vi "GlobalGraphTwo7.vi"(2 "1D Names Input Array":string[](array[string]), 3 "Cluster Array Input":cluster{"Array":dbl[], "Array 2":dbl[]}[](array[cluster]), 4 "Graph Select":dbl, 5 "Function select":string) -> (0 "1D Names Output Array":string[](array[string]), 1 "Cluster Array Output":cluster{"Array":dbl[], "Array 2":dbl[]}[](array[cluster]))   [LabVIEW 2015]
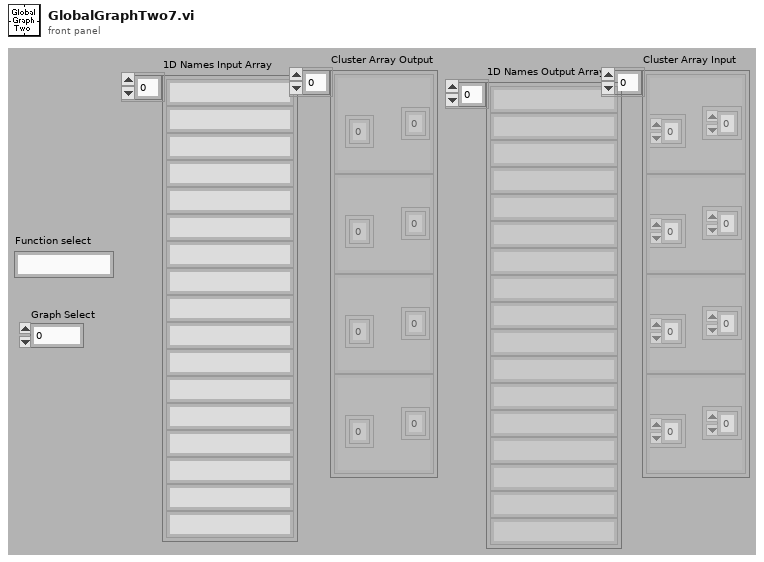
[diagram p1: front panel]
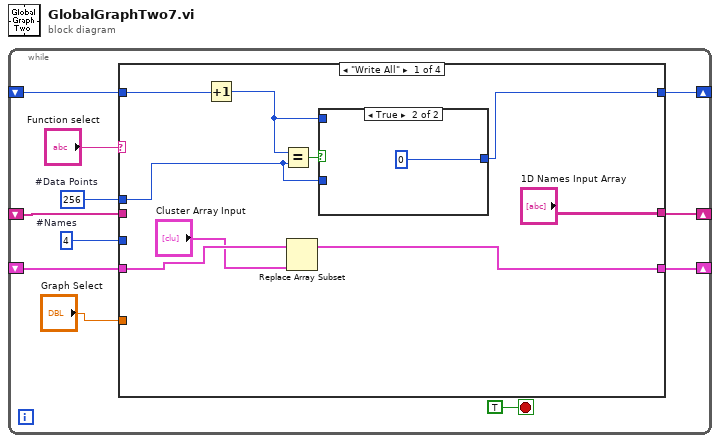
[diagram p0: block diagram]
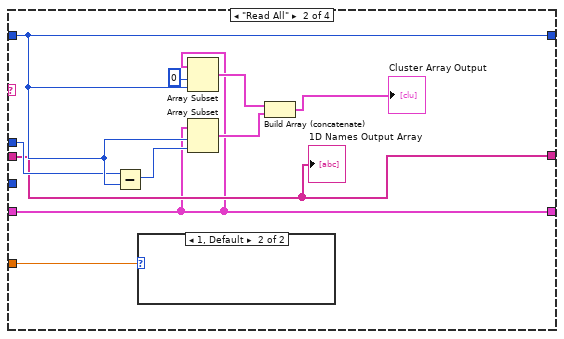
[diagram p3: hidden frame]
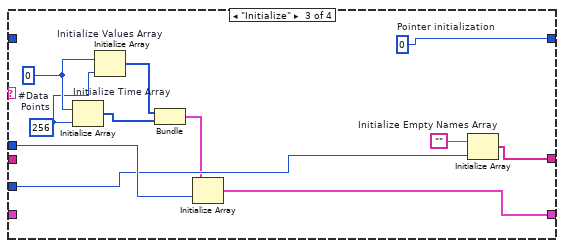
[diagram p5: hidden frame]
diagram:
  n1 = while {
    shift-right: [w9] -> _
    shift-left: _ -> [w7]
    shift-right: [w2] -> _
    shift-left: _ -> [w8]
    shift-right: [w4] -> _
    shift-left: _ -> [w3]
    stop <- TRUE stop-if-true
    w6 = 4  # #Names
    w5 = 256  # #Data Points
    n2 = case shown="\"Write All\"" "Function select" {
      tunnel: [w20 w30 w43 w46] -> w9
      tunnel: w8 -> [w14 w25 _ w45]
      tunnel: w7 -> [w18 w30 _ w46]
      tunnel: w6 -> [_ _ w41 _]
      tunnel: w5 -> [w16 w29 w42 _]
      tunnel: ["1D Names Input Array" w28 w40 w44] -> w4
      tunnel: w3 -> [_ w28 _ w44]
      tunnel: [w13 w25 w34 w45] -> w2
      tunnel: "Graph Select" -> [_ w23 _ _]
      frame "Write All" {
        n3 = Increment(x=w18) -> (x+1=w17:u32)
        n4 = Equal?(x=w17, y=w16) -> (x = y?=w19:bool)
        n5 = Replace Array Subset(array=w14, new element="Cluster Array Input") -> (w13:cluster{i32[], i32[]}[])  [unwired: 1 in]
        n6 = case shown="True" w19 {
          tunnel: [w21 0] -> w20
          tunnel: w17 -> [w21 _]
          tunnel: w16 -> [_ _]
          frame False {
          }
          frame True {
          }
        }
      }
      frame "Read All" {
        n7 = Subtract(x=w29, y=w30) -> (x-y=w31:u32)
        n8 = case shown="1, Default" w23 {
          frame 2 {
          }
          frame 1, Default {
          }
        }
        n9 = Array Subset(array=w25, index=0, length=w30) -> (w27:cluster{i32[], i32[]}[])
        n10 = Array Subset(array=w25, index=w30, length=w31) -> (w26:cluster{i32[], i32[]}[])
        n11 = Build Array (concatenate)(w27, w26) -> (→"Cluster Array Output":cluster{i32[], i32[]}[])
        "1D Names Output Array" <- w28
      }
      frame "Initialize" {
        w38 = 0 ("dimension size")
        w33 = 256  # #Data  Points
        w43 = u32 0  # Pointer initialization
        n12 = Initialize Array "Initialize Time Array"(w38, w33) -> (w36:i32[])
        n13 = Initialize Array "Initialize Values Array"(w38, w33) -> (w37:i32[])
        n14 = Bundle(w37, w36) -> (w35:cluster{i32[], i32[]})  [unwired: 1 in]
        n15 = Initialize Array(w35, w42) -> (w34:cluster{i32[], i32[]}[])
        n16 = Initialize Array "Initialize Empty Names Array"("", w41) -> (w40:string[])
      }
      frame "Read One", Default {
      }
    }
  }
